vi "Idle Control Logic.vi"(8 "error in (no error)":errorcluster, 10 "parameters in":T1, 11 "Sequencer Module runtime in":refnum<class "Sequencer Module runtime.lvclass">) -> (0 "error out":errorcluster, 2 "parameters out":T1, 3 "Sequencer Module runtime out":refnum<class "Sequencer Module runtime.lvclass">)   [LabVIEW 2015, in "Sequencer Module runtime.lvclass"]
doc: "This Vi Controls the Actions Available in the Idle State\nStart New Sequence\nChange Sequence"
uses:
  Sequencer Module runtime.lvclass
  <vilib>/NI/Tag Bus/table/data table.ctl
  Sequencer Module runtime.lvclass/Sequencer Module runtime.ctl
  Sequencer State Enum.ctl
  classes/Step/Execution/StepState.ctl
  classes/Step/Execution/Step State Enum.ctl
  classes/Step/Execution/Step Flow Control.ctl
  classes/Results List/Results List.lvclass
  classes/Step/Execution/Step.lvclass
  classes/Sequence/Execution/Sequence.lvclass
  <vilib>/NI/Tag Bus/table/data table.lvlib
panel:
  # "Manual Input"
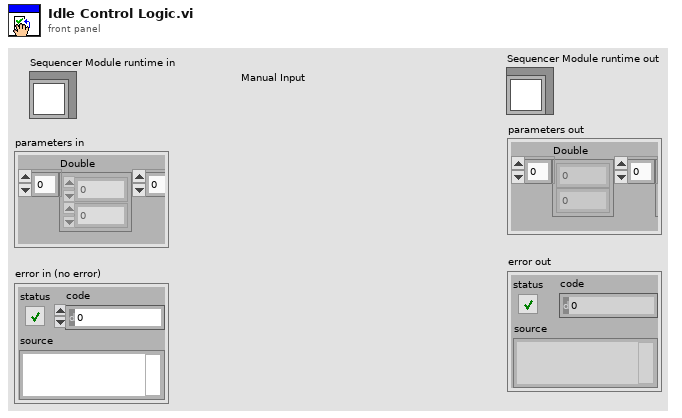
[diagram p1: front panel]
types:
  T1 = typedef "tag bus.lvlib/data table.lvlib/data table.ctl" = cluster{"Double":dbl[], "Single":sgl[], "I64":i64[], "I32":i32[], "I16":i16[], "I8":i8[], "U64":u64[], "U32":u32[], "U16":u16[], "U8":u8[], "Boolean":bool[], "String":string[], "Array of Double":cluster{"DBL Array":dbl[]}[], "Array of Single":cluster{"SGL Array":sgl[]}[], "Array of I64":cluster{"I64 Array":i64[]}[], "Array of I32":cluster{"I32 Array":i32[]}[], "Array of I16":cluster{"I16 Array":i16[]}[], "Array of I8":cluster{"I8 Array":i8[]}[], "Array of U64":cluster{"U64 Array":u64[]}[], "Array of U32":cluster{"U32 Array":u32[]}[], "Array of U16":cluster{"U16 Array":u16[]}[], "Array of U8":cluster{"U8 Array":u8[]}[], "Array of Boolean":cluster{"Boolean Array":bool[]}[], "Array of String":cluster{"String Array":string[]}[]}
  T2 = typedef "Sequencer Module runtime.lvclass/Sequencer Control.ctl" = cluster{"Start":bool, "Change Sequence":bool, "New Sequence":i32, "Pause":bool, "Abort":bool, "Terminate":bool}
  T3 = typedef "Step.lvclass/StepState.ctl" = cluster{"Step State":T4, "Flow Control":T5, "Jump Index":i32, "Done":bool}
  T4 = typedef "Step.lvclass/Step State Enum.ctl" = enum16{"Start", "Skipped", "Timeout", "Completed", "Running", "Aborted"}
  T5 = typedef "Step.lvclass/Step Flow Control.ctl" = enum16{"Next Step", "Jump"}
  T6 = typedef "Sequencer Module runtime.lvclass/Sequencer State Enum.ctl" = enum16{"Idle", "Paused", "Running", "CleanUp", "Generate Report"}
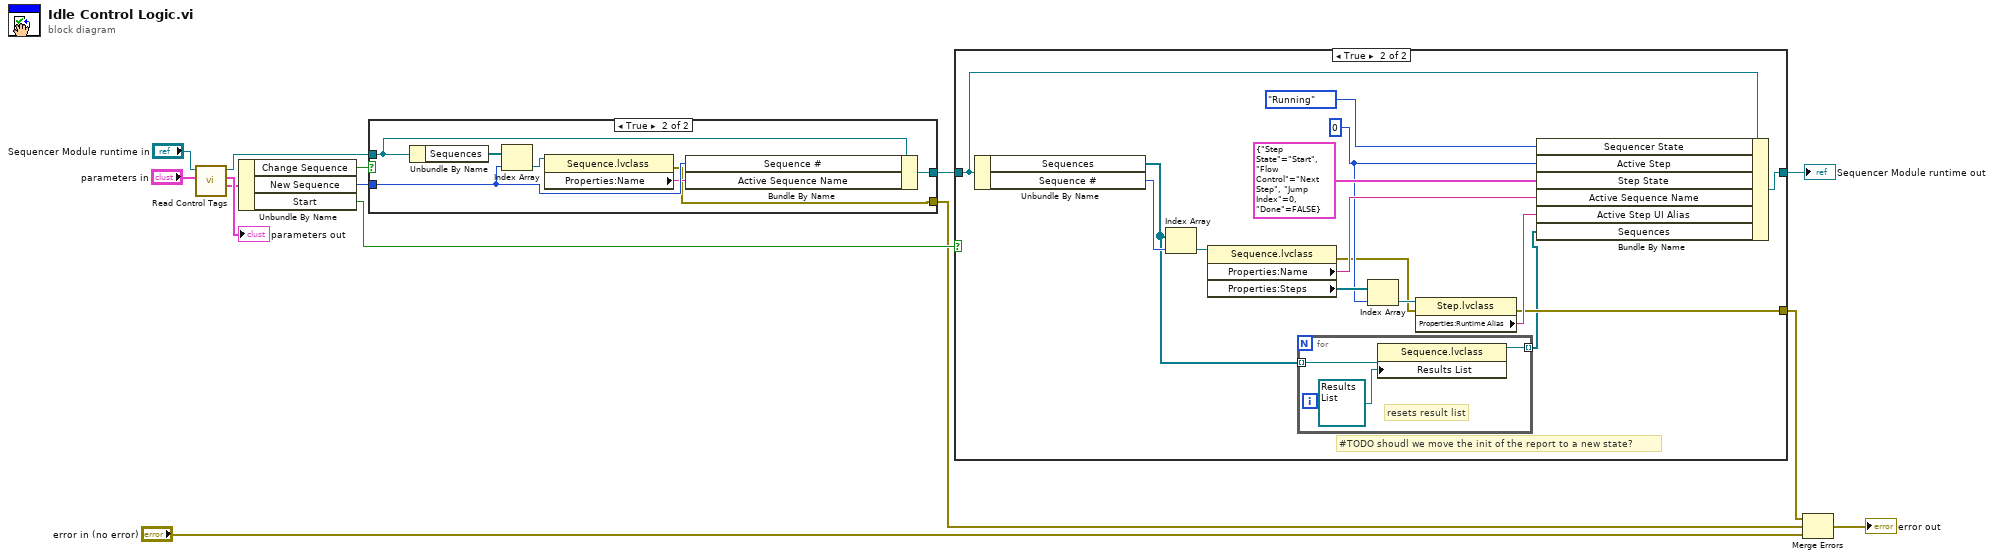
[diagram p0: block diagram]
diagram:
  n1 = call "Read Control Tags.vi"("Paramaters  allocation in"="parameters in", "Sequencer Module runtime in"="Sequencer Module runtime in") -> ("Sequence Control"=w8:T2, "Parameters allocation out"=→"parameters out":T1, "Sequencer Module runtime out"=w4:refnum<class "Sequencer Module runtime.lvclass">)  [unwired: 7 in]
  n2 = Unbundle By Name(w8) -> ("Change Sequence"=w7:bool, "New Sequence"=w6:i32, "Start"=w5:bool)
  n3 = case shown="True" w7 {
    tunnel: w4 -> [w15 w21]
    tunnel: w6 -> [_ w19]
    tunnel: [w15 w22] -> w13
    tunnel: [_ w16] -> w1
    frame False {
    }
    frame True {
      n4 = Unbundle By Name(w21) -> ("Sequences"=w20:refnum<class "Sequence.lvclass">[])
      n5 = Index Array(array=w20, index=w19) -> (element=w18:refnum<class "Sequence.lvclass">)
      n6 = property class="Sequence.lvclass"(reference=w18) -> (error out=w16:errorcluster, "Properties:Name"=w17:string)  [unwired: 1 in, 1 out]
      n7 = Bundle By Name(cluster=w21, "Sequence #"=w19, "Active Sequence Name"=w17) -> (w22:refnum<class "Sequencer Module runtime.lvclass">)
    }
  }
  n8 = case shown="True" w5 {
    tunnel: w13 -> [w23 w34]
    tunnel: [w23 w38] -> w14
    tunnel: [_ w26] -> w2
    frame False {
    }
    frame True {
      w30 = 0 ("Sequencer State.Active Step")
      # "#TODO shoudl we move the init of the report to a new state?"
      n9 = Unbundle By Name(w34) -> ("Sequences"=w25:refnum<class "Sequence.lvclass">[], "Sequence #"=w33:i32)
      n10 = Index Array(array=w25, index=w33) -> (element=w35:refnum<class "Sequence.lvclass">)
      n11 = property class="Sequence.lvclass"(reference=w35) -> (error out=w27:errorcluster, "Properties:Name"=w32:string, "Properties:Steps"=w31:refnum<class "Step.lvclass">[])  [unwired: 1 in, 1 out]
      n12 = for {
        tunnel: w25 -> [w41] mode=indexing
        tunnel: [w39] -> w24 mode=indexing
        # "resets result list"
        n13 = property class="Sequence.lvclass"(reference=w41, "Results List"=refnum<class "Results List.lvclass"> refnum) -> (reference out=w39:refnum<class "Sequence.lvclass">)  [unwired: 1 in, 1 out]
      }
      n14 = Index Array(array=w31, index=w30) -> (element=w29:refnum<class "Step.lvclass">)
      n15 = property class="Step.lvclass"(reference=w29, error in=w27) -> (error out=w26:errorcluster, "Properties:Runtime Alias"=w28:string)  [unwired: 1 out]
      n16 = Bundle By Name(cluster=w34, "Sequencer State"=Sequencer_State_Enum."Running" ("Sequencer State.Sequencer State"), "Active Step"=w30, "Step State"=T3 {"Step State"=enum."Start", "Flow Control"=enum."Next Step", "Jump Index"=0, "Done"=FALSE} ("Sequencer State.Step State"), "Active Sequence Name"=w32, "Active Step UI Alias"=w28, "Sequences"=w24) -> (w38:refnum<class "Sequencer Module runtime.lvclass">)
    }
  }
  "Sequencer Module runtime out" <- w14
  n17 = Merge Errors(w2, w1, "error in (no error)") -> (→"error out":errorcluster)
